vi "ClimbNetwork.vi"   [LabVIEW 2020]
uses:
  ClimbGlobals.vi
  <vilib>/Rock Robotics/Network Tables/NT Write Number.vi
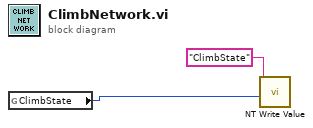
[diagram p0: block diagram]
diagram:
  n1 = global read "ClimbGlobals.vi" "ClimbState"() -> (w1:i32)
  n2 = call-poly <vilib>:"NT Write Value.vi"("Numeric"=w1, "Name"="ClimbState") -> ()  [unwired: 9 in, 1 out]
